vi "Run_EnFlo_Hub.vi"() -> ()   [LabVIEW 2010]
uses:
  Anemometry Sub Vis/Globals/Dynamic_call_global.ph.vi
panel:
  out "No of iterations":i32
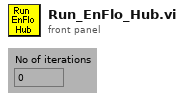
[diagram p1: front panel]
types:
  T1 = enum32{"Bad", "Idle", "Run top level", "Running"}
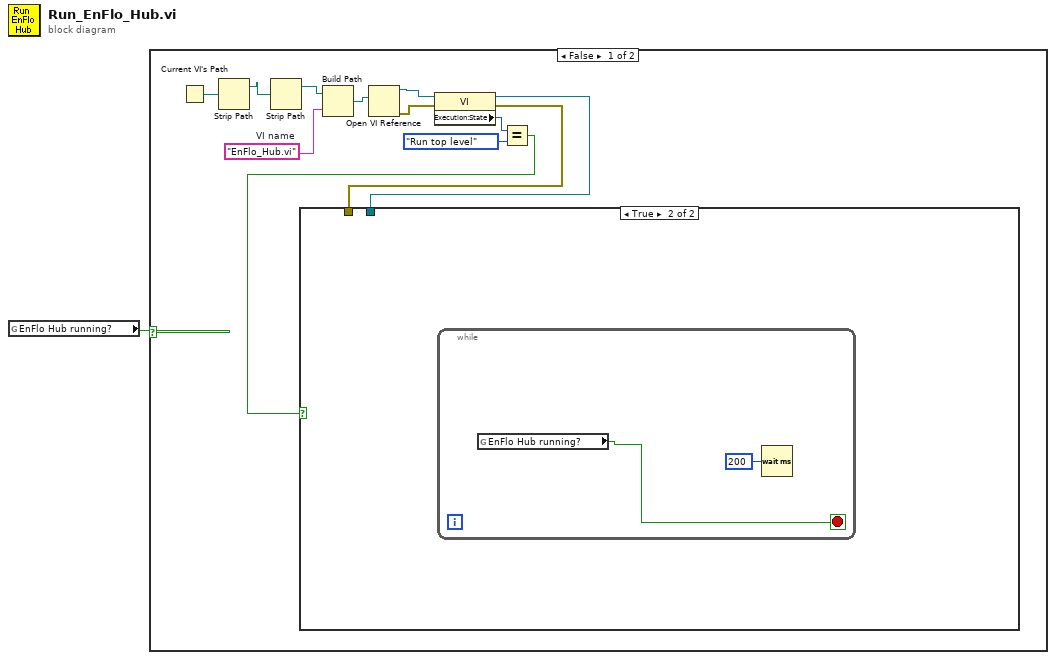
[diagram p0: block diagram]
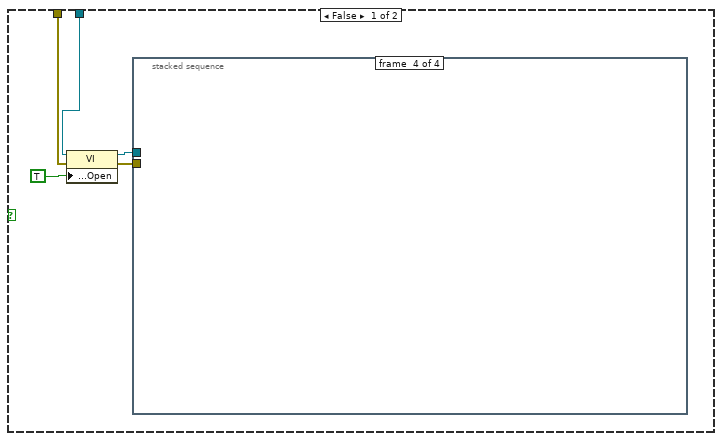
[diagram p2: hidden frame]
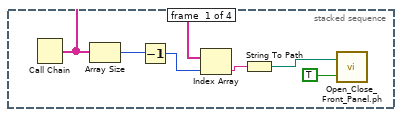
[diagram p3: hidden frame]
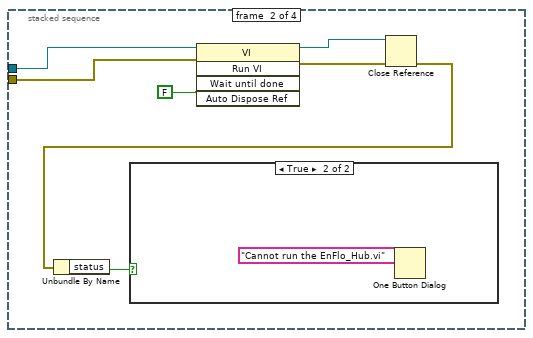
[diagram p4: hidden frame]
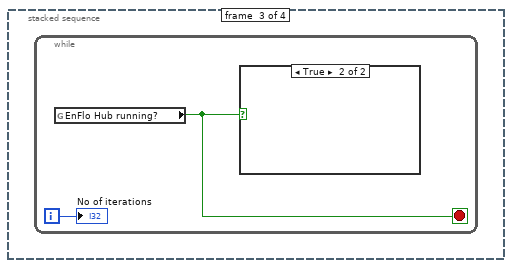
[diagram p6: hidden frame]
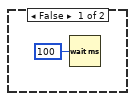
[diagram p7: hidden frame]
diagram:
  n1 = global read "Dynamic_call_global.ph.vi" "EnFlo Hub running?"() -> (w1:bool)
  n2 = case shown="False" w1 {
    frame False {
      w8 = "EnFlo_Hub.vi"  # VI name
      n3 = Current VI's Path() -> (path=w7:path)
      n4 = Strip Path(path=w7) -> (stripped path=w9:path)  [unwired: 1 out]
      n5 = Strip Path(path=w9) -> (stripped path=w10:path)  [unwired: 1 out]
      n6 = Build Path(base path=w10, name or relative path=w8) -> (appended path=w13:path)
      n7 = Open VI Reference(vi path=w13) -> (vi reference=w11:refnum<vi>, error out=w12:errorcluster)  [unwired: 2 in, 3 out]
      n8 = property class="VI"(reference=w11, error in=w12) -> (reference out=w2:refnum<vi>, error out=w3:errorcluster, "Execution:State"=w6:T1)
      n9 = Equal?(x=w6, y=T1."Run top level" ("Execution:State")) -> (x = y?=w4:bool)
      n10 = case shown="True" w4 {
        tunnel: w3 -> [w17 _]
        tunnel: w2 -> [w16 _]
        frame False {
          n11 = property class="VI"(reference=w16, error in=w17, "Front Panel Window:Open"=TRUE) -> (reference out=w15:refnum<vi>, error out=w14:errorcluster)
          n12 = stacked-sequence {
            tunnel: w15 -> [_ w26 _ _]
            tunnel: w14 -> [_ w25 _ _]
            frame #0 {
              n13 = Call Chain() -> (call chain=w19:string[])
              n14 = Array Size(array=w19) -> (size(s)=w24:i32)
              n15 = Decrement(x=w24) -> (x-1=w23:i32)
              n16 = Index Array(array=w19, index=w23) -> (element=w22:string)
              n17 = String To Path(string=w22) -> (path=w21:path)
              n18 = call "Open_Close_Front_Panel.ph.vi"("Front Panel Window:Open"=TRUE, "VI path"=w21) -> ()  [unwired: 2 out]
            }
            frame #1 {
              w31 = FALSE ("Wait until done")
              n19 = invoke class="VI" method="Run VI"(reference=w26, error in=w25, "Wait until done"=w31, "Auto Dispose Ref"=w31) -> (reference out=w30:refnum<vi>, error out=w29:errorcluster)  [unwired: 1 in, 3 out]
              n20 = Close Reference(reference=w30, error in (no error)=w29) -> (error out=w28:errorcluster)
              n21 = Unbundle By Name(w28) -> ("status"=w27:bool)
              n22 = case shown="True" w27 {
                frame False {
                }
                frame True {
                  n23 = One Button Dialog(message="Cannot run the EnFlo_Hub.vi") -> ()  [unwired: 2 out]
                }
              }
            }
            frame #2 {
              n24 = while {
                i -> [w33]
                stop <- w34 stop-if-true
                n25 = global read "Dynamic_call_global.ph.vi" "EnFlo Hub running?"() -> (w34:bool)
                n26 = case shown="True" w34 {
                  frame False {
                    n27 = Wait (ms)(milliseconds to wait=u32 100) -> ()  [unwired: 1 out]
                  }
                  frame True {
                  }
                }
                "No of iterations" <- w33
              }
            }
            frame #3 {
            }
          }
        }
        frame True {
          n28 = while {
            stop <- w37 stop-if-true
            n29 = global read "Dynamic_call_global.ph.vi" "EnFlo Hub running?"() -> (w37:bool)
            n30 = Wait (ms)(milliseconds to wait=u32 200) -> ()  [unwired: 1 out]
          }
        }
      }
    }
    frame True {
    }
  }
